vi "AutoStacking V1.0.vi"(10 "Abort":bool, 11 "Tote Button":bool) -> (2 "Number Totes":dbl, 3 "Finished":bool)   [LabVIEW 2014]
uses:
  Autostacking State.ctl
panel:
  out "Autostacking State 2":T1
  in  "Autostacking State":T1
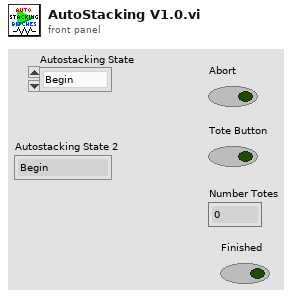
[diagram p1: front panel]
types:
  T1 = typedef "Autostacking State.ctl" = enum16{"Begin", "Bottom", "Middle", "Wait", "Done", "Abort"}
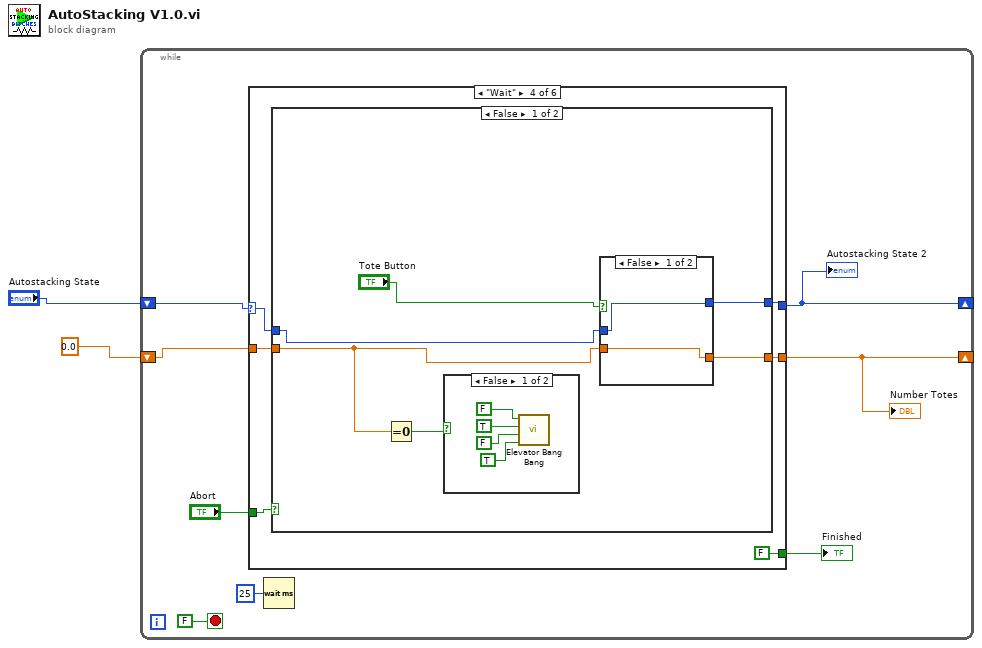
[diagram p0: block diagram]
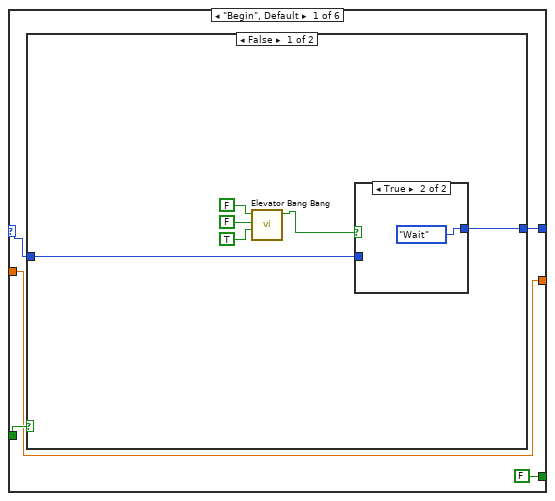
[diagram p2: hidden frame]
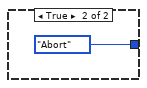
[diagram p4: hidden frame]
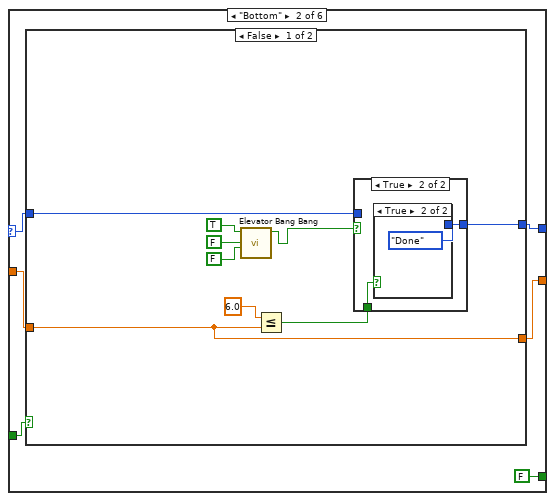
[diagram p5: hidden frame]
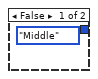
[diagram p7: hidden frame]
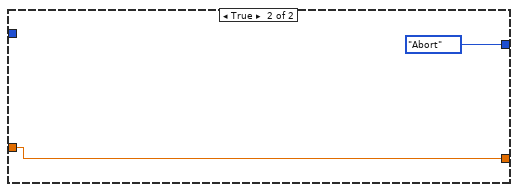
[diagram p8: hidden frame]
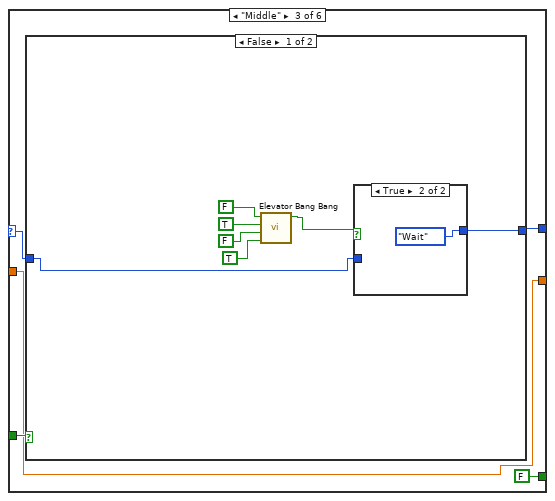
[diagram p9: hidden frame]
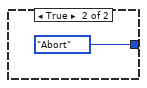
[diagram p11: hidden frame]
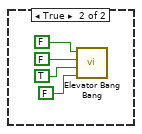
[diagram p12: hidden frame]
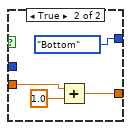
[diagram p13: hidden frame]
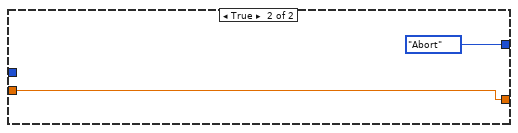
[diagram p14: hidden frame]
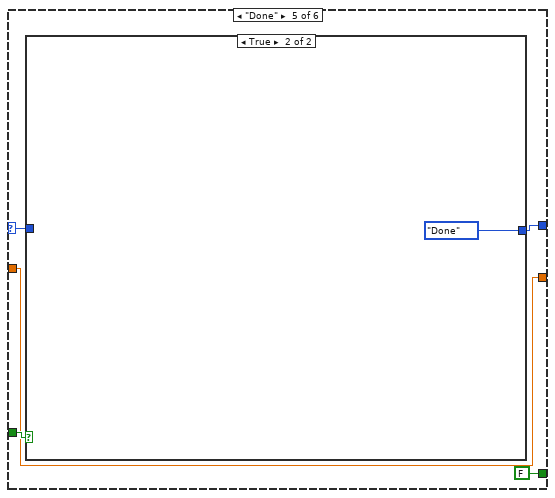
[diagram p15: hidden frame]
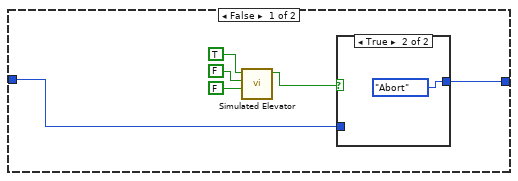
[diagram p16: hidden frame]
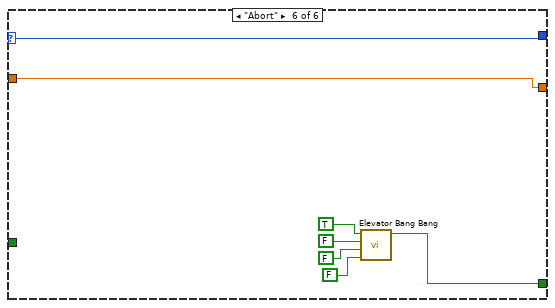
[diagram p18: hidden frame]
diagram:
  n1 = while {
    shift-right: [w6] -> _
    shift-left: "Autostacking State" -> [w10]
    shift-right: [w4] -> _
    shift-left: 0.0 -> [w5]
    stop <- FALSE stop-if-true
    n2 = case shown="\"Wait\"" w10 {
      selector: w10 -> [w13 w28 w49 w67 w92 w110]
      tunnel: "Abort" -> [w15 w30 w51 w65 w94 _]
      tunnel: [w14 w29 w50 w66 w93 w110] -> w6
      tunnel: [w12 w26 w48 w64 w91 w109] -> w4
      tunnel: w5 -> [w12 w27 w48 w63 w91 w109]
      tunnel: [FALSE FALSE FALSE FALSE FALSE w104] -> w3
      frame "Begin", Default {
        n3 = case shown="False" w15 {
          tunnel: [w21 Autostacking_State."Abort" ("Autostacking State")] -> w14
          tunnel: w13 -> [w20 _]
          frame False {
            n4 = call "Elevator Bang Bang.vi"("Top"=TRUE, "Middle"=FALSE, "Bottom"=FALSE) -> ("in range"=w16:bool)  [unwired: 8 in]
            n5 = case shown="True" w16 {
              tunnel: [w22 Autostacking_State."Wait" ("Autostacking State")] -> w21
              tunnel: w20 -> [w22 _]
              frame False {
              }
              frame True {
              }
            }
          }
          frame True {
          }
        }
      }
      frame "Bottom" {
        n6 = case shown="False" w30 {
          tunnel: [w39 Autostacking_State."Abort" ("Autostacking State")] -> w29
          tunnel: w28 -> [w38 _]
          tunnel: w27 -> [w36 w45]
          tunnel: [w36 w45] -> w26
          frame False {
            n7 = call "Elevator Bang Bang.vi"("Top"=FALSE, "Middle"=FALSE, "Bottom"=TRUE) -> ("in range"=w31:bool)  [unwired: 8 in]
            n8 = Less Or Equal?(x=6.0, y=w36) -> (x <= y?=w35:bool)
            n9 = case shown="True" w31 {
              tunnel: [w40 w42] -> w39
              tunnel: w38 -> [w40 _]
              tunnel: w35 -> [_ w41]
              frame False {
              }
              frame True {
                n10 = case shown="True" w41 {
                  tunnel: [Autostacking_State."Middle" ("Autostacking State") Autostacking_State."Done" ("Autostacking State")] -> w42
                  frame False {
                  }
                  frame True {
                  }
                }
              }
            }
          }
          frame True {
          }
        }
      }
      frame "Middle" {
        n11 = case shown="False" w51 {
          tunnel: [w58 Autostacking_State."Abort" ("Autostacking State")] -> w50
          tunnel: w49 -> [w57 _]
          frame False {
            n12 = call "Elevator Bang Bang.vi"("Hold Up Mode"=TRUE, "Top"=FALSE, "Middle"=TRUE, "Bottom"=FALSE) -> ("in range"=w52:bool)  [unwired: 7 in]
            n13 = case shown="True" w52 {
              tunnel: [w59 Autostacking_State."Wait" ("Autostacking State")] -> w58
              tunnel: w57 -> [w59 _]
              frame False {
              }
              frame True {
              }
            }
          }
          frame True {
          }
        }
      }
      frame "Wait" {
        n14 = case shown="False" w65 {
          tunnel: [w73 Autostacking_State."Abort" ("Autostacking State")] -> w66
          tunnel: w67 -> [w72 _]
          tunnel: [w71 w88] -> w64
          tunnel: w63 -> [w69 w88]
          frame False {
            n15 = Equal To 0?(x=w69) -> (x = 0?=w70:bool)
            n16 = case shown="False" w70 {
              frame False {
                n17 = call "Elevator Bang Bang.vi"("Hold Up Mode"=TRUE, "Top"=FALSE, "Middle"=TRUE, "Bottom"=FALSE) -> ()  [unwired: 7 in, 1 out]
              }
              frame True {
                n18 = call "Elevator Bang Bang.vi"("Hold Up Mode"=FALSE, "Top"=TRUE, "Middle"=FALSE, "Bottom"=FALSE) -> ()  [unwired: 7 in, 1 out]
              }
            }
            n19 = case shown="False" "Tote Button" {
              tunnel: [w83 Autostacking_State."Bottom" ("Autostacking State")] -> w73
              tunnel: w72 -> [w83 _]
              tunnel: [w82 w85] -> w71
              tunnel: w69 -> [w82 w84]
              frame False {
              }
              frame True {
                n20 = Add(x=w84, y=1.0) -> (x+y=w85:dbl)
              }
            }
          }
          frame True {
          }
        }
      }
      frame "Done" {
        n21 = case shown="True" w94 {
          tunnel: [w100 Autostacking_State."Done" ("Autostacking State")] -> w93
          tunnel: w92 -> [w99 _]
          frame False {
            n22 = call "Simulated Elevator.vi"("Top"=FALSE, "Middle"=FALSE, "Bottom"=TRUE) -> ("in Range"=w98:bool)  [unwired: 8 in]
            n23 = case shown="True" w98 {
              tunnel: [w101 Autostacking_State."Abort" ("Autostacking State")] -> w100
              tunnel: w99 -> [w101 _]
              frame False {
              }
              frame True {
              }
            }
          }
          frame True {
          }
        }
      }
      frame "Abort" {
        n24 = call "Elevator Bang Bang.vi"("Hold Up Mode"=FALSE, "Top"=FALSE, "Middle"=FALSE, "Bottom"=TRUE) -> ("in range"=w104:bool)  [unwired: 7 in]
      }
    }
    "Autostacking State 2" <- w6
    "Number Totes" <- w4
    "Finished" <- w3
    n25 = Wait (ms)(milliseconds to wait=u32 25) -> ()  [unwired: 1 out]
  }
